vi "MICSD Serial Read.vi"(7 "Timeout(mS)":dbl=3000.0, 8 "error in (no error)":errorcluster, 11 "VISA Resource Name":refnum<visa-resource-name>) -> (0 "error out":errorcluster, 2 "Read Data":u8[](array[numeric]), 3 "DUP Visa Resource Name":refnum<visa-resource-name>)   [LabVIEW 2020]
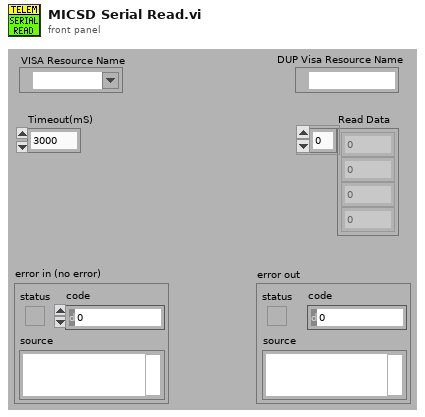
[diagram p1: front panel]
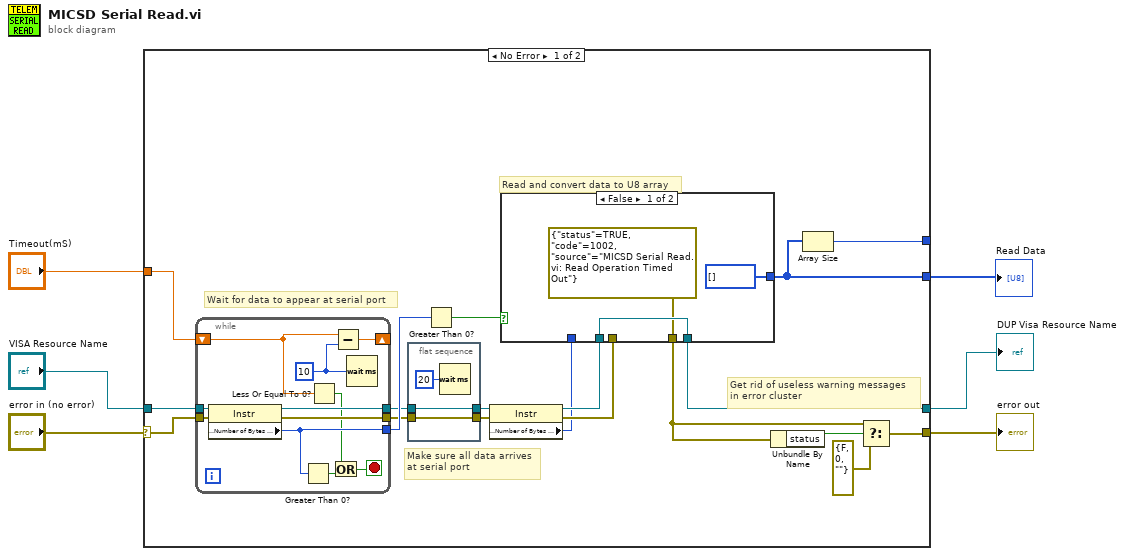
[diagram p0: block diagram]
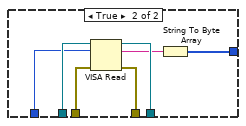
[diagram p2: hidden frame]
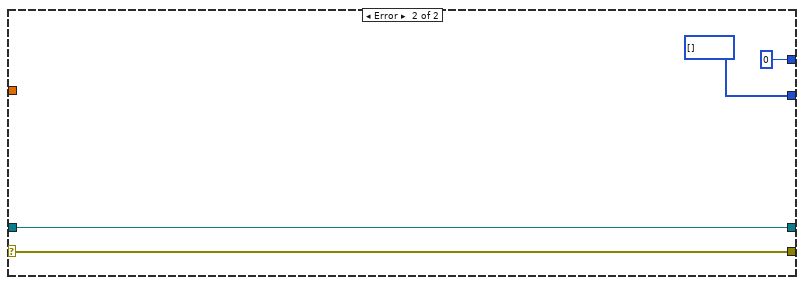
[diagram p3: hidden frame]
diagram:
  n1 = case shown="No Error" "error in (no error)" {
    selector: "error in (no error)" -> [w22 w52]
    tunnel: "VISA Resource Name" -> [w23 w53]
    tunnel: [w24 w53] -> w4
    tunnel: [w16 w52] -> w3
    tunnel: [w10 u8[] []] -> w2
    tunnel: "Timeout(mS)" -> [w20 _]
    tunnel: [w9 0] -> _
    frame No Error {
      # "Make sure all data arrives\nat serial port"
      # "Read and convert data to U8 array"
      # "Wait for data to appear at serial port"
      # "Get rid of useless warning messages\nin error cluster"
      n2 = while {
        tunnel: [w39] -> w8
        tunnel: [w38] -> w12
        tunnel: w23 -> [w37]
        tunnel: w22 -> [w36]
        tunnel: [w34] -> w21
        shift-right: [w35] -> _
        shift-left: w20 -> [w30]
        stop <- w32 stop-if-true
        w31 = u32 10 ("milliseconds to wait")
        n3 = property class="Instr"(reference=w37, error in=w36) -> (reference out=w39:refnum<visa-resource-name>, error out=w38:errorcluster, "Serial Settings:Number of Bytes at Serial Port"=w34:u32)
        n4 = Greater Than 0?(x=w34) -> (x > 0?=w33:bool)
        n5 = Less Or Equal To 0?(x=w30) -> (x <= 0?=w29:bool)
        n6 = Or(x=w29, y=w33) -> (x .or. y?=w32:bool)
        n7 = Subtract(x=w30, y=w31) -> (x-y=w35:dbl)
        n8 = Wait (ms)(milliseconds to wait=w31) -> ()  [unwired: 1 out]
      }
      n9 = flat-sequence {
        tunnel: w12 -> [w28]
        tunnel: [w28] -> w11
        tunnel: w8 -> [w26]
        tunnel: [w26] -> w7
        frame #0 {
          n10 = Wait (ms)(milliseconds to wait=u32 20) -> ()  [unwired: 1 out]
        }
      }
      n11 = Greater Than 0?(x=w21) -> (x > 0?=w25:bool)
      n12 = property class="Instr"(reference=w7, error in=w11) -> (reference out=w19:refnum<visa-resource-name>, error out=w18:errorcluster, "Serial Settings:Number of Bytes at Serial Port"=w17:u32)
      n13 = case shown="False" w25 {
        tunnel: w18 -> [_ w49]
        tunnel: w19 -> [w42 w48]
        tunnel: [errorcluster {"status"=TRUE, "code"=1002, "source"="MICSD Serial Read.vi: Read Operation Timed Out"} ("error out") w47] -> w15
        tunnel: [w42 w46] -> w24
        tunnel: [u8[] [] w43] -> w10
        tunnel: w17 -> [_ w45]
        frame False {
        }
        frame True {
          n14 = VISA Read(VISA resource name=w48, byte count=w45, error in (no error)=w49) -> (VISA resource name out=w46:refnum<visa-resource-name>, read buffer=w44:string, error out=w47:errorcluster)  [unwired: 1 out]
          n15 = String To Byte Array(string=w44) -> (unsigned byte array=w43:u8[])
        }
      }
      n16 = Unbundle By Name(w15) -> ("status"=w14:bool)
      n17 = Array Size(array=w10) -> (size(s)=w9:i32)
      n18 = Select(t=w15, s=w14, f=errorcluster {"status"=FALSE, "code"=0, "source"=""} ("error out")) -> (s? t:f=w16:errorcluster)
    }
    frame Error {
    }
  }
  "DUP Visa Resource Name" <- w4
  "error out" <- w3
  "Read Data" <- w2
